vi "DriveReadEncoder.vi"(8 "error in":errorcluster, 11 "ModualNamePrefix":i32) -> (0 "error out":errorcluster, 2 "SWERVE_DRIVE_MODULE_POSITION":T1={"Distance"=0.0, "Angle"={"VALUE"=0.0, "COS"=1.0, "SIN"=0.0}, "P"=FALSE} {"Angle"."SIN" format="%13.4f"; "Angle"."COS" format="%13.4f"; "Angle"."VALUE" format="%13.4f"}, 3 "SWERVE_DRIVE_MODULE_STATE":T3={"Speed"=0.0, "Angle"={"VALUE"=0.0, "COS"=1.0, "SIN"=0.0}} {"Angle"."SIN" format="%13.4f"; "Angle"."COS" format="%13.4f"; "Angle"."VALUE" format="%13.4f"})   [LabVIEW 2023]
uses:
  <vilib>/Rock Robotics/WPI/ThirdParty/JAS_Junk/TrajLib/TypeDef/SWERVE_DRIVE_MODULE_STATE.ctl
  <vilib>/Rock Robotics/WPI/ThirdParty/JAS_Junk/TrajLib/TypeDef/ROTATION2D.ctl
  <vilib>/Rock Robotics/WPI/ThirdParty/JAS_Junk/TrajLib/TypeDef/SWERVE_DRIVE_MODULE_POSITION.ctl
  <vilib>/Rock Robotics/WPI/ThirdParty/JAS_Junk/TrajLib/Conv_Deg_Radians.vi
  <vilib>/Rock Robotics/WPI/ThirdParty/JAS_Junk/TrajLib/Rotation2d_CreateAngle.vi
  DriveGlobal.vi
  <vilib>/Rock Robotics/WPI/ThirdParty/Phoenix-LabVIEW/CANCoder/CTRE_Phoenix_CANcoder_RefNumRegistryGet.vi
  <vilib>/Rock Robotics/WPI/MotorControl/WPI_MotorControlRefNum Registry Get.vi
  <vilib>/Rock Robotics/WPI/ThirdParty/Phoenix-LabVIEW/CANCoder/Get/CTRE_Phoenix_CANcoder_GetSensorData.vi
  <vilib>/Rock Robotics/Network Tables/NT Write Number.vi
  <vilib>/Rock Robotics/WPI/ThirdParty/JAS_Junk/TrajLib/Trajectory_Library.lvlib
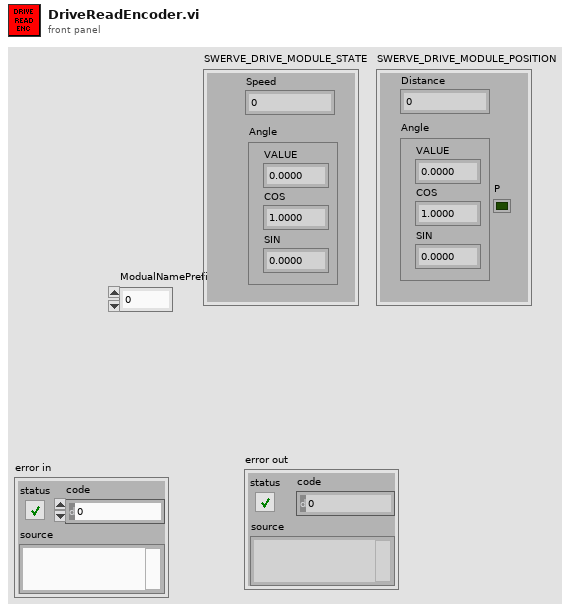
[diagram p1: front panel]
types:
  T1 = typedef "Trajectory_Library.lvlib/SWERVE_DRIVE_MODULE_POSITION.ctl" = cluster{"Distance":dbl, "Angle":T2, "P":bool}
  T2 = typedef "Trajectory_Library.lvlib/ROTATION2D.ctl" = cluster{"VALUE":dbl, "COS":dbl, "SIN":dbl}
  T3 = typedef "Trajectory_Library.lvlib/SWERVE_DRIVE_MODULE_STATE.ctl" = cluster{"Speed":dbl, "Angle":T2}
  T4 = typedef "WPI_MotorControlDeviceRef.ctl" = cluster{"DeviceStatus":errorcluster, "Type":T5, "PWM":cluster{"PWM Channel":T6, "DeadBand":T7}, "CAN":cluster{"Device Number":u8, "SetOutput VI Ref":variant, "GetOutput VI Ref":variant, "Enable VI Ref":variant, "Disable VI Ref":variant, "Data":variant}, "Invert":bool, "DIO PWM":cluster{"PWM \"Enable\" Channel":T6, "DIOChannel":T8, "PWM Rate":dbl}}
  T5 = typedef "WPI_MotorControlType.ctl" = enum16{"PWM", "CAN", "DIO PWM"}
  T6 = typedef "FPGA_DIOPWMChannel.ctl" = enum8{"PWM 0", "PWM 1", "PWM 2", "PWM 3", "PWM 4", "PWM 5", "PWM 6", "PWM 7", "PWM 8", "PWM 9", "PWM MXP 0", "PWM MXP 1", "PWM MXP 2", "PWM MXP 3", "PWM MXP 4", "PWM MXP 5", "PWM MXP 6", "PWM MXP 7", "PWM MXP 8", "PWM MXP 9", "Invalid"}
  T7 = typedef "WPI_PWMDeadband.ctl" = cluster{"Name":string, "maxPositivePwm":i32, "minPositivePwm":i32, "centerPwm":i32, "maxNegativePwm":i32, "minNegativePwm":i32, "angularRange":u16}
  T8 = typedef "FPGA_DIOChannel.ctl" = enum8{"DIO 0", "DIO 1", "DIO 2", "DIO 3", "DIO 4", "DIO 5", "DIO 6", "DIO 7", "DIO 8", "DIO 9", "DIO MXP 0", "DIO MXP 1", "DIO MXP 2", "DIO MXP 3", "DIO MXP 4", "DIO MXP 5", "DIO MXP 6", "DIO MXP 7", "DIO MXP 8", "DIO MXP 9", "DIO MXP 10", "DIO MXP 11", "DIO MXP 12", "DIO MXP 13", "DIO MXP 14", "DIO MXP 15", "SPI Port CS1", "SPI Port CS2", "SPI Port CS3", "SPI Port MISO", "SPI Port MOSI", "Invalid"}
  T9 = typedef "CTRE_Phoenix_CANcoder_DeviceRef.ctl" = cluster{"DeviceStatus":errorcluster, "Device Number":u8, "Handle":u64, "UsageFrame":u32, "Library Path":path}
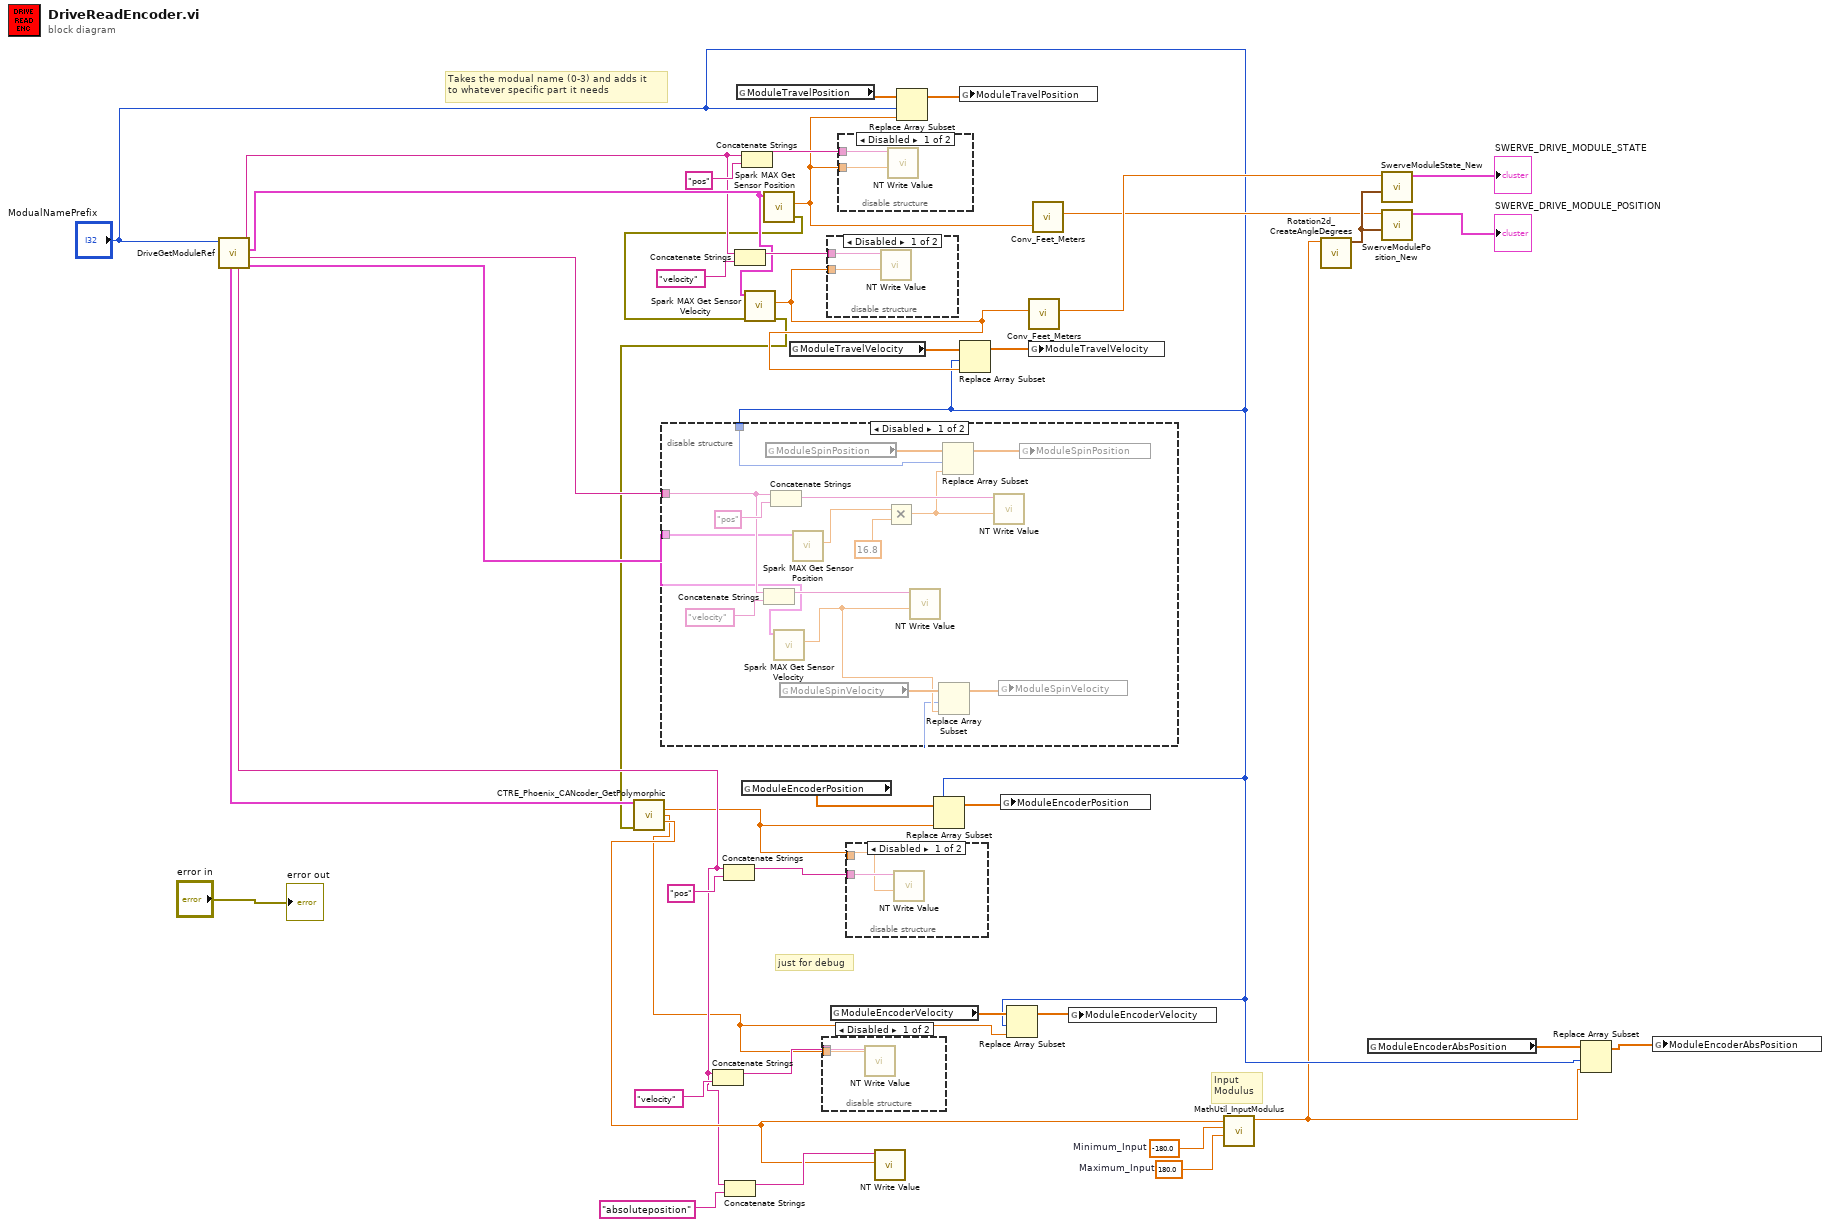
[diagram p0: block diagram]
diagram:
  w29 = -180.0  # Minimum_Input
  w28 = 180.0  # Maximum_Input
  # "Input\nModulus"
  # "just for debug"
  # "Takes the modual name (0-3) and adds it \nto whatever specific part it needs"
  n1 = call "DriveGetModuleRef.vi"("ModualNamePrefix"="ModualNamePrefix") -> ("SpinMot"=w19:T4, "SpinStr"=w21:string, "TravMot"=w33:T4, "TravStr"=w20:string, "EncStr"=w18:string, "EncDevice"=w17:T9)  [unwired: 5 in]
  n2 = disable-structure shown="Disabled" {
    disable-tunnel: w21 -> [w52 _]
    disable-tunnel: w19 -> [w51 _]
    disable-tunnel: "ModualNamePrefix" -> [w44 _]
    frame Disabled {
      n3 = Concatenate Strings(w52, "velocity" ("refnum name")) -> (w55:string)
      n4 = global read "DriveGlobal.vi" "ModuleSpinPosition"() -> (w50:dbl[])
      n5 = Concatenate Strings(w52, "pos" ("refnum name")) -> (w57:string)
      n6 = call <vilib>:"Spark MAX Get Sensor Velocity.vi"("MotorControlDevRef in"=w51) -> ("Sensor Velocity"=w45:dbl)  [unwired: 7 in, 3 out]
      n7 = global read "DriveGlobal.vi" "ModuleSpinVelocity"() -> (w47:dbl[])
      n8 = call <vilib>:"Spark MAX Get Sensor Position.vi"("MotorControlDevRef in"=w51) -> ("Sensor Position"=w54:dbl)  [unwired: 7 in, 3 out]
      n9 = Multiply(x=w54, y=16.8) -> (x*y=w48:dbl)
      n10 = call-poly <vilib>:"NT Write Value.vi"("value"=w45, "name"=w55) -> ()  [unwired: 9 in, 1 out]
      n11 = Replace Array Subset(array=w47, new element=w45, index=w44) -> (w46:dbl[])
      n12 = Replace Array Subset(array=w50, new element=w48, index=w44) -> (w49:dbl[])
      n13 = call-poly <vilib>:"NT Write Value.vi"("value"=w48, "name"=w57) -> ()  [unwired: 9 in, 1 out]
      n14 = global write "DriveGlobal.vi" "ModuleSpinVelocity"(w46) -> ()
      n15 = global write "DriveGlobal.vi" "ModuleSpinPosition"(w49) -> ()
    }
    frame Enabled {
    }
  }
  n16 = Concatenate Strings(w18, "velocity" ("refnum name")) -> (w40:string)
  n17 = Concatenate Strings(w18, "pos" ("refnum name")) -> (w42:string)
  n18 = Concatenate Strings(w18, "absoluteposition" ("refnum name")) -> (w38:string)
  n19 = Concatenate Strings(w20, "velocity" ("refnum name")) -> (w34:string)
  n20 = global read "DriveGlobal.vi" "ModuleTravelPosition"() -> (w24:dbl[])
  n21 = Concatenate Strings(w20, "pos" ("refnum name")) -> (w36:string)
  n22 = global read "DriveGlobal.vi" "ModuleEncoderPosition"() -> (w13:dbl[])
  n23 = call <vilib>:"Spark MAX Get Sensor Position.vi"("MotorControlDevRef in"=w33) -> ("error out"=w3:errorcluster, "Sensor Position"=w22:dbl)  [unwired: 7 in, 2 out]
  n24 = call <vilib>:"Spark MAX Get Sensor Velocity.vi"("error in (no error)"=w3, "MotorControlDevRef in"=w33) -> ("error out"=w2:errorcluster, "Sensor Velocity"=w14:dbl)  [unwired: 6 in, 2 out]
  n25 = call-poly <vilib>:"CTRE_Phoenix_CANcoder_GetPolymorphic.vi"("CTRE_CANcoder_DeviceRef"=w17, "error in"=w2) -> ("Position"=w11:dbl, "Velocity"=w8:dbl, "Absolute Position"=w27:dbl)  [unwired: 9 in, 2 out]
  n26 = global read "DriveGlobal.vi" "ModuleTravelVelocity"() -> (w16:dbl[])
  n27 = disable-structure shown="Disabled" {
    disable-tunnel: w40 -> [w60 _]
    disable-tunnel: w8 -> [w59 _]
    frame Disabled {
      n28 = call-poly <vilib>:"NT Write Value.vi"("value"=w59, "name"=w60) -> ()  [unwired: 9 in, 1 out]
    }
    frame Enabled {
    }
  }
  n29 = disable-structure shown="Disabled" {
    disable-tunnel: w34 -> [w62 _]
    disable-tunnel: w14 -> [w61 _]
    frame Disabled {
      n30 = call-poly <vilib>:"NT Write Value.vi"("value"=w61, "name"=w62) -> ()  [unwired: 9 in, 1 out]
    }
    frame Enabled {
    }
  }
  n31 = global read "DriveGlobal.vi" "ModuleEncoderVelocity"() -> (w10:dbl[])
  n32 = disable-structure shown="Disabled" {
    disable-tunnel: w36 -> [w64 _]
    disable-tunnel: w22 -> [w63 _]
    frame Disabled {
      n33 = call-poly <vilib>:"NT Write Value.vi"("value"=w63, "name"=w64) -> ()  [unwired: 9 in, 1 out]
    }
    frame Enabled {
    }
  }
  n34 = disable-structure shown="Disabled" {
    disable-tunnel: w42 -> [w66 _]
    disable-tunnel: w11 -> [w65 _]
    frame Disabled {
      n35 = call-poly <vilib>:"NT Write Value.vi"("value"=w65, "name"=w66) -> ()  [unwired: 9 in, 1 out]
    }
    frame Enabled {
    }
  }
  n36 = call-poly <vilib>:"NT Write Value.vi"("value"=w27, "name"=w38) -> ()  [unwired: 9 in, 1 out]
  n37 = Replace Array Subset(array=w24, new element=w22, index="ModualNamePrefix") -> (w23:dbl[])
  n38 = Replace Array Subset(array=w13, new element=w11, index="ModualNamePrefix") -> (w12:dbl[])
  n39 = global write "DriveGlobal.vi" "ModuleTravelPosition"(w23) -> ()
  n40 = Replace Array Subset(array=w16, new element=w14, index="ModualNamePrefix") -> (w15:dbl[])
  n41 = global write "DriveGlobal.vi" "ModuleEncoderPosition"(w12) -> ()
  n42 = Replace Array Subset(array=w10, new element=w8, index="ModualNamePrefix") -> (w9:dbl[])
  n43 = call <vilib>:"Conv_Feet_Meters.vi"("Feet"=w14) -> ("Meters"=w26:dbl)  [unwired: 10 in]
  n44 = global write "DriveGlobal.vi" "ModuleTravelVelocity"(w15) -> ()
  n45 = call <vilib>:"Conv_Feet_Meters.vi"("Feet"=w22) -> ("Meters"=w25:dbl)  [unwired: 10 in]
  n46 = global write "DriveGlobal.vi" "ModuleEncoderVelocity"(w9) -> ()
  n47 = call <vilib>:"MathUtil_InputModulus.vi"("Maximum_Input"=w28, "Minimum_Input"=w29, "Input"=w27) -> ("modulus"=w4:dbl)  [unwired: 8 in]
  n48 = call <vilib>:"Rotation2d_CreateAngleDegrees.vi"("Angle_Degrees"=w4) -> ("ROTATION"=w32:T2)  [unwired: 10 in]
  n49 = global read "DriveGlobal.vi" "ModuleEncoderAbsPosition"() -> (w7:dbl[])
  n50 = call <vilib>:"SwerveModuleState_New.vi"("ROTATION"=w32, "Speed"=w26) -> ("SWERVE_DRIVE_MODULE_STATE"=→"SWERVE_DRIVE_MODULE_STATE":T3)  [unwired: 9 in]
  n51 = call <vilib>:"SwerveModulePosition_New.vi"("ROTATION"=w32, "Distance"=w25) -> ("SWERVE_DRIVE_MODULE_POSITION"=→"SWERVE_DRIVE_MODULE_POSITION":T1)  [unwired: 9 in]
  n52 = Replace Array Subset(array=w7, new element=w4, index="ModualNamePrefix") -> (w6:dbl[])
  n53 = global write "DriveGlobal.vi" "ModuleEncoderAbsPosition"(w6) -> ()
  "error out" <- "error in"
